vi "Initialize Modbus Client TCP.vi"(5 "timeout, ms (300)":u32=300, 6 "station address (255)":u8=255, 7 "protocol (TCP)":enum16{"RTU", "ASCII", "TCP"}(ring)=enum."TCP", 8 "error in (no error)":errorcluster, 9 "port (502)":u16=502, 10 "ip address":string, 11 "MODBUS in":refnum<class "PL Modbus Client.lvclass">) -> (0 "error out":errorcluster, 3 "MODBUS out":refnum<class "PL Modbus Client.lvclass">)   [LabVIEW 2015, in "PL Modbus Client.lvclass"]
doc: "Initializes TCP connection to Modbus server using specified settings."
uses:
  PL Modbus Client.lvclass
  PL Modbus Client.lvclass/PL Modbus Client.ctl
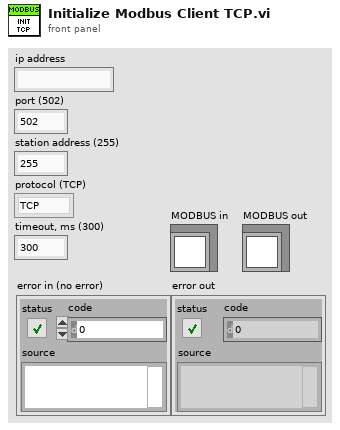
[diagram p1: front panel]
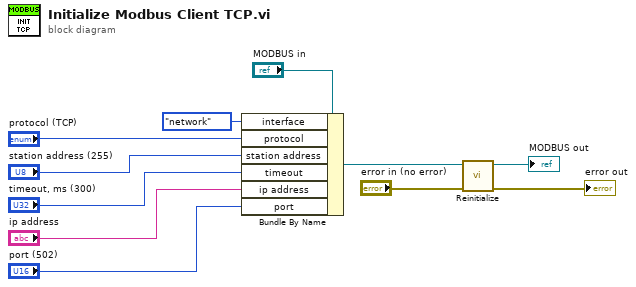
[diagram p0: block diagram]
diagram:
  n1 = Bundle By Name(cluster="MODBUS in", "interface"=enum16{"serial", "network"}."network", "protocol"="protocol (TCP)", "station address"="station address (255)", "timeout"="timeout, ms (300)", "ip address"="ip address", "port"="port (502)") -> (w10:refnum<class "PL Modbus Client.lvclass">)
  n2 = call "Reinitialize.vi"("error in (no error)"="error in (no error)", "MODBUS in"=w10) -> ("error out"=→"error out":errorcluster, "MODBUS out"=→"MODBUS out":refnum<class "PL Modbus Client.lvclass">)  [unwired: 8 in]
